vi "6_Eon.vi"(0 "file path (IN)":path, 1 "VGE":dbl, 2 "VCE":dbl, 5 "Project #":string, 7 "Request #":string, 9 "TEST #":string, 11 "error in (no error)":errorcluster) -> (4 "file path (OUT)":path, 6 "ON Region":waveform(dbl)[](graph) caption="Eon (uj)", 8 "Eon (uj)":dbl, 10 "DONE Eon":bool, 15 "error out":errorcluster)   [LabVIEW 2020]
uses:
  <vilib>/Waveform/WDTOps.llb/WDT Waveform Duration DBL.vi
  <vilib>/Waveform/WDTOps.llb/WDT Get Waveform Subset DBL.vi
  <vilib>/measure/mascope.llb/Transition Measurements 1 chan.vi
  <vilib>/measure/NI_MAPro.lvlib
panel:
  in  "Decision ?":bool
  in  "Cursor a : Channel 3\nfall edge tolerance":dbl=0.1
  in  "Cursor a : Channel 3\nfall edge number":i32=1 min=1
  in  "Cursor a : Channel 2\nrise edge tolerance":dbl=0.1
  in  "Cursor a : Channel 2\nrise edge number":i32=1 min=1
  out "Cursor a : Channel 2":dbl
  out "Cursor a : Channel 3":dbl
  out "Eon : XY Graph":cluster{"X":dbl, "Y":dbl}[](graph)
  out "Eon Area Y-axis":dbl[](array[numeric])
  out "Eon Area X-axis":dbl[](array[numeric])
  out "3% Vce":dbl
  out "10% Vge":dbl
  out "measurement info (CH3)":T1 {"ref levels"."ref units" items=["absolute", "relative"]; "ref levels"."high ref level" format="%.2p"; "ref levels"."low ref level" format="%.2p"; "ref levels"."mid ref level" format="%.2p"; "end time" format="%.6e"; "start time" format="%.6e"}
  out "measurement info (CH2)":T1 {"ref levels"."ref units" items=["absolute", "relative"]; "ref levels"."high ref level" format="%.2p"; "ref levels"."low ref level" format="%.2p"; "ref levels"."mid ref level" format="%.2p"; "end time" format="%.6e"; "start time" format="%.6e"}
  in  "reference  levels (CH2 initialize)":T2={"high ref level"=90.0, "mid ref level"=50.0, "low ref level"=10.0, "ref units"=1} {"ref units" items=["absolute", "percent"]; "high ref level" format="%0.2f"; "low ref level" format="%0.2f"; "mid ref level" format="%0.2f"}
  in  "reference  levels (CH3 initialize)":T2={"high ref level"=90.0, "mid ref level"=50.0, "low ref level"=10.0, "ref units"=1} {"ref units" items=["absolute", "percent"]; "high ref level" format="%0.2f"; "low ref level" format="%0.2f"; "mid ref level" format="%0.2f"}
  out "Waveform Graph":waveform(dbl)[](graph)
  # "From 10% Vge to 3% Vce"
  # "Default = 1"
  # "Default = 1"
  # "Default = 0.1"
  # "Default = 0.1"
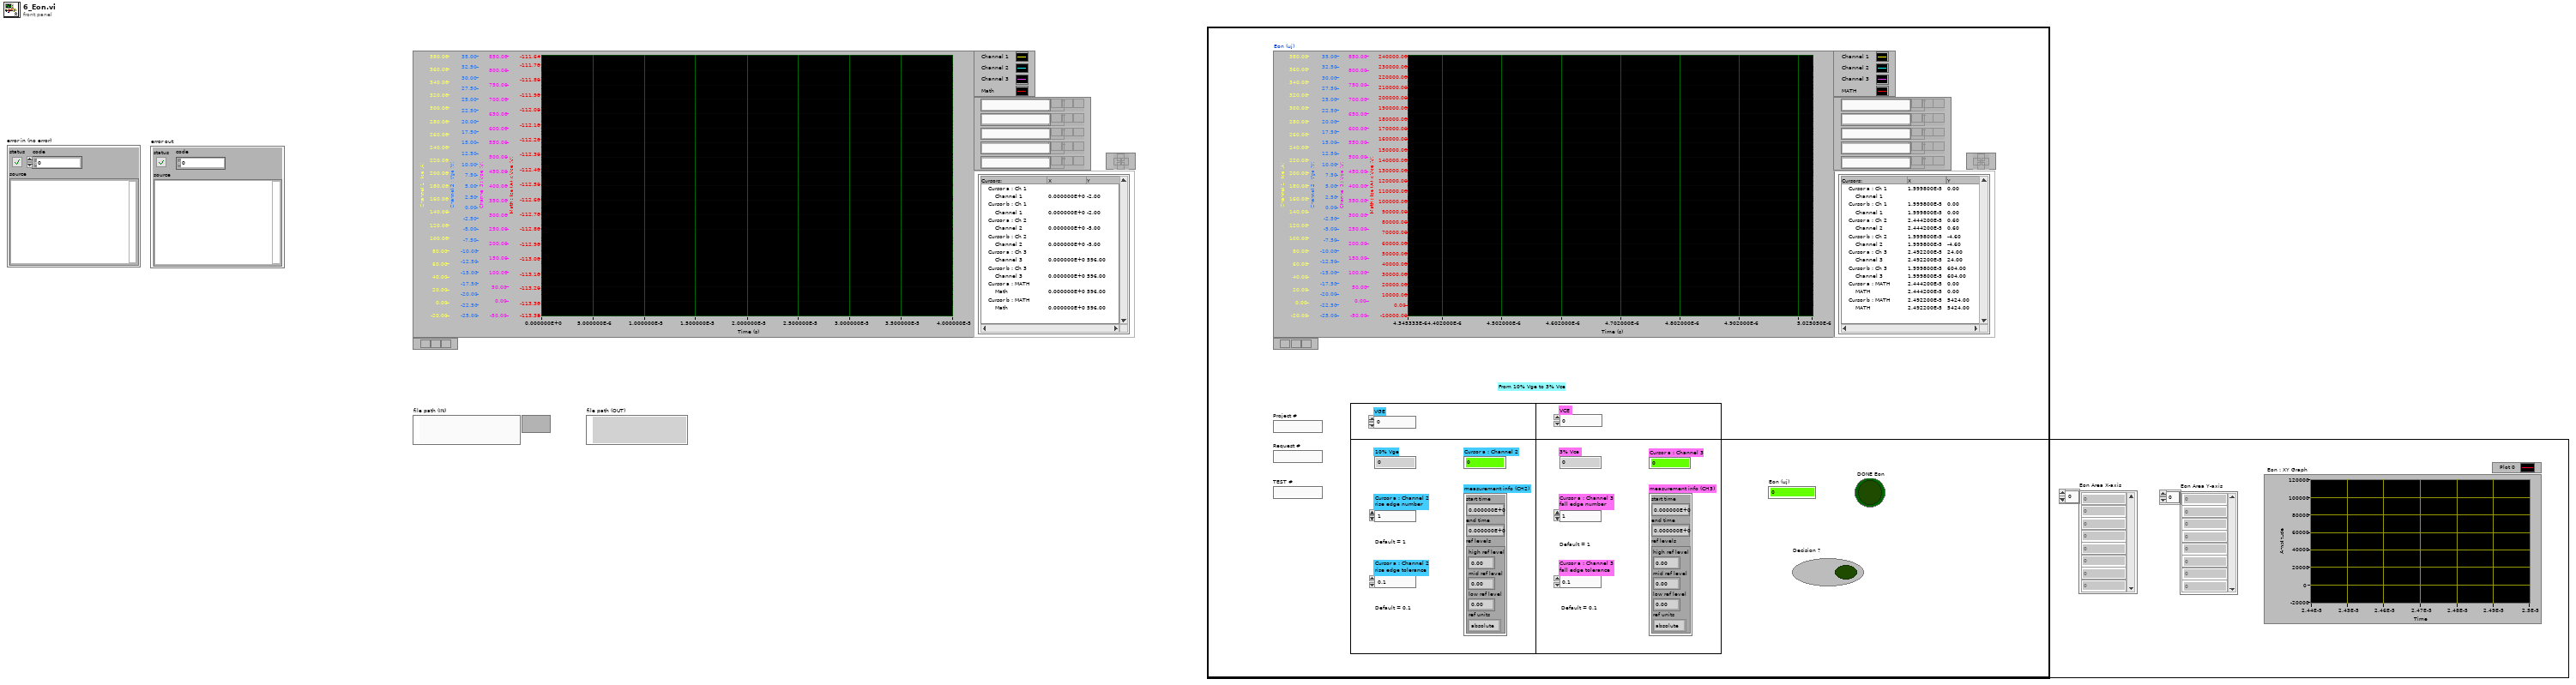
[diagram p1: front panel]
types:
  T1 = cluster{"start time":dbl, "end time":dbl, "ref levels":cluster{"high ref level":dbl, "mid ref level":dbl, "low ref level":dbl, "ref units":u16}}
  T2 = cluster{"high ref level":dbl, "mid ref level":dbl, "low ref level":dbl, "ref units":u16}
  T3 = enum32{"Invalid", "Standard", "Closed", "Hidden", "Minimized", "Maximized"}
  T4 = typedef "imagedata.ctl" = cluster{"image type":i32, "image depth":i32, "image":u8[], "mask":u8[], "colors":u32[], "Rectangle":cluster{"left":i16, "top":i16, "right":i16, "bottom":i16}}
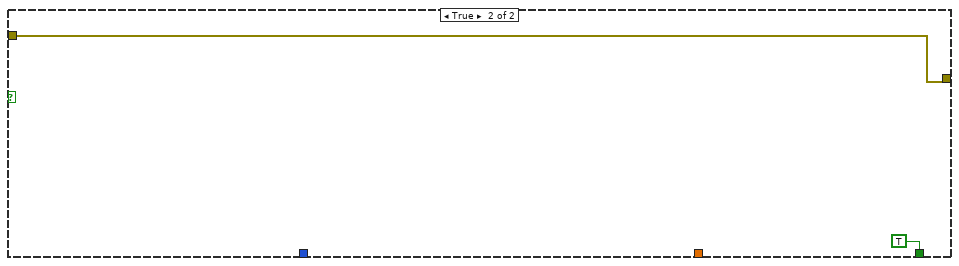
[diagram p6: hidden frame]
diagram:
  w7 = 0.0 ("Eon (uj)")
  w16 = errorcluster {"status"=FALSE, "code"=0, "source"=""} ("error out")
  w8 = FALSE ("DONE Tdon")
  w17 = waveform(dbl)[] [] ("Waveform Graph")
  n1 = local write "Eon (uj)"(w7) -> ()
  n2 = local write "Cursor a : Channel 2"(w7) -> ()
  n3 = local write "Cursor a : Channel 3"(w7) -> ()
  n4 = local write "Cursor a : Channel 2\nrise edge tolerance"(0.1 ("Cursor a : Channel 2\nrise edge tolerance")) -> ()
  n5 = local write "Cursor a : Channel 2\nrise edge number"(1 ("Cursor a : Channel 2\nrise edge number")) -> ()
  n6 = local write "DONE Eon"(w8) -> ()
  n7 = local write "Cursor a : Channel 3\nfall edge tolerance"(0.1 ("Cursor a : Channel 3\nfall edge tolerance")) -> ()
  n8 = local write "Cursor a : Channel 3\nfall edge number"(1 ("Cursor a : Channel 3\nfall edge number")) -> ()
  n9 = local write "Decision ?"(w8) -> ()
  n10 = local write "error out"(w16) -> ()
  n11 = local write "error in (no error)"(w16) -> ()
  n12 = local write "Waveform Graph"(w17) -> ()
  n13 = local write "ON Region"(w17) -> ()
  n14 = disable-structure shown="Disabled" {
    frame Disabled {
      n15 = control-ref of="This VI"() -> (w19:refnum<vi>)
      n16 = invoke class="VI" method="FP.Close"() -> (reference=w18:refnum<vi>)  [unwired: 2 in, 3 out]
      n17 = invoke class="VI" method="FP.Open"(reference=w19, "Activate"=TRUE ("Activate?"), "State"=T3."Maximized") -> (error in=w22:errorcluster, error out=w20:errorcluster)  [unwired: 1 in, 4 out]
      n18 = property class="VI"(reference=w19, error in=w20, "Front Panel.Closeable"=TRUE ("Front Panel Window:Closeable")) -> ()  [unwired: 2 out]
    }
    frame Enabled {
    }
  }
  n19 = flat-sequence {
    tunnel: ["file path (IN)"] -> w6
    tunnel: [w25] -> w5
    tunnel: [w36] -> w12
    tunnel: [w35] -> w9
    tunnel: w6 -> [w34]
    tunnel: w5 -> [w33]
    tunnel: w12 -> [w388]
    tunnel: [w387] -> w11
    tunnel: [w386] -> w10
    tunnel: w9 -> [w386]
    tunnel: w11 -> [w401]
    tunnel: w10 -> [w402]
    frame #0 {
      n20 = control-ref of="This VI"() -> (w27:refnum<vi>)
      n21 = invoke class="VI" method="FP.Open"(reference=w27, error in="error in (no error)", "Activate"=TRUE ("Activate?"), "State"=T3."Maximized") -> (error out=w28:errorcluster)  [unwired: 1 in, 4 out]
      n22 = property class="VI"(reference=w27, error in=w28, "Front Panel.Closeable"=TRUE ("Front Panel Window:Closeable")) -> (error out=w25:errorcluster)  [unwired: 1 out]
    }
    frame #1 {
      n23 = while {
        shift-right: [w43] -> w36
        shift-left: w33 -> [w41]
        tunnel: [w39] -> w35
        tunnel: w34 -> [w38]
        stop <- w44 stop-if-true
        n24 = flat-sequence {
          tunnel: w41 -> [w85]
          tunnel: [w85] -> w42
          tunnel: w38 -> [w78]
          tunnel: [w78] -> w37
          tunnel: [w117] -> w70
          tunnel: [w104] -> w69
          tunnel: [w115] -> w68
          tunnel: [w105] -> w67
          tunnel: [w87] -> w66
          tunnel: w42 -> [w191]
          tunnel: w37 -> [w186]
          tunnel: w70 -> [w231]
          tunnel: w69 -> [w230]
          tunnel: w68 -> [w229]
          tunnel: [w217] -> w65
          tunnel: w67 -> [w216]
          tunnel: [w216] -> w64
          tunnel: [w213] -> w63
          tunnel: [w212] -> w62
          tunnel: w66 -> [w211]
          tunnel: [w211] -> w61
          tunnel: w65 -> [w261]
          tunnel: [w258] -> w60
          tunnel: w64 -> [w267]
          tunnel: [w267] -> w59
          tunnel: w63 -> [w266]
          tunnel: [w266] -> w58
          tunnel: w62 -> [w265]
          tunnel: [w265] -> w57
          tunnel: w61 -> [w264]
          tunnel: [w264] -> w56
          tunnel: w60 -> [w278]
          tunnel: [w273] -> w55
          tunnel: w59 -> [w279]
          tunnel: [w279] -> w54
          tunnel: w58 -> [w269]
          tunnel: [w269] -> w53
          tunnel: w57 -> [w270]
          tunnel: [w270] -> w52
          tunnel: w56 -> [w277]
          tunnel: w55 -> [w360]
          tunnel: [w359] -> w51
          tunnel: w54 -> [w367]
          tunnel: [w367] -> w50
          tunnel: w53 -> [w356]
          tunnel: w52 -> [w355]
          tunnel: [w355] -> w49
          tunnel: [w356] -> w48
          tunnel: w51 -> [w378]
          tunnel: [w377] -> w47
          tunnel: w50 -> [w379]
          tunnel: [w379] -> w46
          tunnel: w49 -> [w372]
          tunnel: w48 -> [w371]
          tunnel: w47 -> [w382]
          tunnel: w46 -> [w380]
          tunnel: [w381] -> w45
          tunnel: [w380] -> w39
          frame #0 {
            w84 = waveform(dbl)[] [] ("Waveform Graph")
            w80 = 0.0 ("Eon (uj)")
            w79 = FALSE ("DONE Tdon")
            n25 = local write "Eon (uj)"(w80) -> ()
            n26 = local write "Cursor a : Channel 2"(w80) -> ()
            n27 = local write "Cursor a : Channel 3"(w80) -> ()
            n28 = local write "DONE Eon"(w79) -> ()
            n29 = local write "Decision ?"(w79) -> ()
            n30 = local write "Eon Area X-axis"(dbl[] [] ("Eon Area X-axis")) -> ()
            n31 = local write "Eon : XY Graph"(cluster{"X":dbl, "Y":dbl}[] [] ("Eon : XY Graph")) -> ()
            n32 = local write "Eon Area Y-axis"(dbl[] [] ("Eon Area X-axis")) -> ()
            n33 = Wait (ms)(milliseconds to wait=u32 200) -> ()  [unwired: 1 out]
            n34 = local write "Waveform Graph"(w84) -> ()
            n35 = local write "ON Region"(w84) -> ()
          }
          frame #1 {
            w94 = u16 1 items=["Samples", "Relative Time"] ("start/duration format")
            w168 = u16 1 items=["Samples", "Relative Time"] ("start/duration format")
            w178 = u16 1 items=["Samples", "Relative Time"] ("start/duration format")
            w179 = u16 1 items=["Samples", "Relative Time"] ("start/duration format")
            # "Channel 3"
            # "Channel 1"
            # "Channel MATH"
            # "MATH = Ch1 x Ch3"
            # "Channel 1"
            # "Channel 3"
            # "Channel 2"
            # "dt"
            # "Ch2"
            # "Ch1"
            n36 = call "3_ReadDatatoWaveform.vi"("error in (no error)"=w191, "file path (IN)"=w186) -> ("error out"=w164:errorcluster, "Waveform Graph"=→"Waveform Graph":waveform(dbl)[], "file path (OUT)"=w105:path, "dt"=w187:dbl, "Ch 2 Data"=w184:dbl[], "Ch 3 Data"=w188:dbl[], "Ch 1 Data"=w185:dbl[])  [unwired: 3 in]
            n37 = call <vilib>:"Beep.vi"("use system alert? (T)"=FALSE, "duration (msec)"=u32 200, "frequency (Hz)"=u32 2000) -> ()  [unwired: 9 in]
            n38 = To Time Stamp(1:0.0 ("number")) -> (0:w189:timestamp)
            n39 = disable-structure shown="Enabled" {
              disable-tunnel: w189 -> [w206 _]
              disable-tunnel: w187 -> [w205 _]
              disable-tunnel: w188 -> [w204 _]
              disable-tunnel: [w203 _] -> w101
              frame Enabled {
                # "Channel 3"
                n40 = Bundle By Name("Y"=w204, "dt"=w205, "t0"=w206) -> (w203:waveform(dbl))  [unwired: 1 in]
              }
              frame Disabled {
              }
            }
            n41 = disable-structure shown="Enabled" {
              disable-tunnel: w189 -> [w202 _]
              disable-tunnel: w187 -> [w201 _]
              disable-tunnel: w184 -> [w200 _]
              disable-tunnel: [w199 _] -> w167
              frame Enabled {
                # "Channel 2"
                n42 = Bundle By Name("Y"=w200, "dt"=w201, "t0"=w202) -> (w199:waveform(dbl))  [unwired: 1 in]
              }
              frame Disabled {
              }
            }
            n43 = disable-structure shown="Enabled" {
              disable-tunnel: w189 -> [w198 _]
              disable-tunnel: w187 -> [w197 _]
              disable-tunnel: w185 -> [w196 _]
              disable-tunnel: [w195 _] -> w102
              frame Enabled {
                # "Channel 1"
                n44 = Bundle By Name("Y"=w196, "dt"=w197, "t0"=w198) -> (w195:waveform(dbl))  [unwired: 1 in]
              }
              frame Disabled {
              }
            }
            n45 = Unbundle By Name(w101) -> ("Y"=w98:dbl[])
            n46 = Unbundle By Name(w102) -> ("Y"=w99:dbl[], "dt"=w86:dbl, "t0"=w100:timestamp)
            n47 = for {
              tunnel: w99 -> [w194] mode=indexing
              tunnel: w98 -> [w193] mode=indexing
              tunnel: [w192] -> w97 mode=indexing
              n48 = Multiply(x=w194, y=w193) -> (x*y=w192:dbl)
            }
            n49 = Bundle By Name("Y"=w97, "dt"=w86, "t0"=w100) -> (w89:waveform(dbl))  [unwired: 1 in]
            n50 = call-poly <vilib>:"Waveform Duration.vi"("waveform in"=w89) -> ("error out"=w90:errorcluster, "duration"=w92:dbl, "waveform out"=w95:waveform(dbl))  [unwired: 8 in]
            n51 = call-poly <vilib>:"Waveform Duration.vi"("error in (no error)"=w164, "waveform in"=w101) -> ("error out"=w172:errorcluster, "duration"=w170:dbl, "waveform out"=w103:waveform(dbl))  [unwired: 7 in]
            n52 = call-poly <vilib>:"Waveform Duration.vi"("error in (no error)"=w164, "waveform in"=w167) -> ("error out"=w173:errorcluster, "duration"=w176:dbl, "waveform out"=w174:waveform(dbl))  [unwired: 7 in]
            n53 = call-poly <vilib>:"Waveform Duration.vi"("error in (no error)"=w164, "waveform in"=w102) -> ("error out"=w183:errorcluster, "duration"=w180:dbl, "waveform out"=w182:waveform(dbl))  [unwired: 7 in]
            n54 = Divide(x=w92, y=2.0) -> (x/y=w93:dbl)
            n55 = Divide(x=w170, y=2.0) -> (x/y=w169:dbl)
            n56 = Divide(x=w176, y=2.0) -> (x/y=w177:dbl)
            n57 = Divide(x=w180, y=2.0) -> (x/y=w165:dbl)
            n58 = call-poly <vilib>:"Get Waveform Subset.vi"("start/duration format"=w94, "error in (no error)"=w90, "duration"=w93, "start samples/time"=w93, "waveform in"=w95) -> ("error out"=w88:errorcluster, "waveform out"=w87:waveform(dbl))  [unwired: 1 in, 2 out]
            n59 = call-poly <vilib>:"Get Waveform Subset.vi"("start/duration format"=w168, "error in (no error)"=w172, "duration"=w169, "start samples/time"=w169, "waveform in"=w103) -> ("error out"=w161:errorcluster, "waveform out"=w104:waveform(dbl))  [unwired: 1 in, 2 out]
            n60 = call-poly <vilib>:"Get Waveform Subset.vi"("start/duration format"=w178, "error in (no error)"=w173, "duration"=w177, "start samples/time"=w177, "waveform in"=w174) -> ("error out"=w162:errorcluster, "waveform out"=w117:waveform(dbl))  [unwired: 1 in, 2 out]
            n61 = call-poly <vilib>:"Get Waveform Subset.vi"("start/duration format"=w179, "error in (no error)"=w183, "duration"=w165, "start samples/time"=w165, "waveform in"=w182) -> ("error out"=w163:errorcluster, "waveform out"=w116:waveform(dbl))  [unwired: 1 in, 2 out]
            n62 = Build Array(w116, w117, w104, w87) -> (→"ON Region":waveform(dbl)[])
            n63 = Merge Errors(w163, w162, w161, w88) -> (w113:errorcluster)
            n64 = property on="ON Region" class="WFGraph (strict)"(error in=w113) -> (error out=w112:errorcluster, "Width"=w111:u32)  [unwired: 1 in, 1 out]
            n65 = property on="ON Region" class="WFGraph (strict)"(error in=w112, "Caption.Justify"=enum16{"Left", "Center", "Right"}."Left" ("Caption.Justification"), "Caption.Width"=w111, "Caption.FontBold"=TRUE ("Caption.Font:Bold"), "Caption.FontColor"=u32 16860 ("Caption.Font:Color"), "Caption.FontSize"=u32 24 ("Caption.Font:Size"), "Caption.Text"="Eon (uj)") -> (error out=w107:errorcluster)  [unwired: 1 in, 1 out]
            n66 = property on="ON Region" class="WFGraph (strict)"(error in=w107, "XScale.Offset"=w165) -> (error out=w141:errorcluster)  [unwired: 1 in, 1 out]
            n67 = property on="ON Region" class="WFGraph (strict)"(error in=w141, "Active Cursor"=u32 0, "Cursor.Cursor X"=0.0 ("Cursor.Cursor Position:Cursor X"), "Cursor.Cursor Y"=0.0 ("Cursor.Cursor Position:Cursor Y"), "Cursor.Visible"=FALSE) -> (error out=w140:errorcluster)  [unwired: 1 in, 1 out]
            n68 = property on="ON Region" class="WFGraph (strict)"(error in=w140, "Active Cursor"=u32 1, "Cursor.Cursor X"=0.0 ("Cursor.Cursor Position:Cursor X"), "Cursor.Cursor Y"=0.0 ("Cursor.Cursor Position:Cursor Y"), "Cursor.Visible"=FALSE) -> (error out=w139:errorcluster)  [unwired: 1 in, 1 out]
            n69 = property on="ON Region" class="WFGraph (strict)"(error in=w139, "Active Cursor"=u32 2, "Cursor.Cursor X"=0.0 ("Cursor.Cursor Position:Cursor X"), "Cursor.Cursor Y"=0.0 ("Cursor.Cursor Position:Cursor Y"), "Cursor.Visible"=FALSE) -> (error out=w138:errorcluster)  [unwired: 1 in, 1 out]
            n70 = property on="ON Region" class="WFGraph (strict)"(error in=w138, "Active Cursor"=u32 3, "Cursor.Cursor X"=0.0 ("Cursor.Cursor Position:Cursor X"), "Cursor.Cursor Y"=0.0 ("Cursor.Cursor Position:Cursor Y"), "Cursor.Visible"=FALSE) -> (error out=w121:errorcluster)  [unwired: 1 in, 1 out]
            n71 = property on="ON Region" class="WFGraph (strict)"(error in=w121, "Active Cursor"=u32 4, "Cursor.Cursor X"=0.0 ("Cursor.Cursor Position:Cursor X"), "Cursor.Cursor Y"=0.0 ("Cursor.Cursor Position:Cursor Y"), "Cursor.Visible"=FALSE) -> (error out=w120:errorcluster)  [unwired: 1 in, 1 out]
            n72 = property on="ON Region" class="WFGraph (strict)"(error in=w120, "Active Cursor"=u32 5, "Cursor.Cursor X"=0.0 ("Cursor.Cursor Position:Cursor X"), "Cursor.Cursor Y"=0.0 ("Cursor.Cursor Position:Cursor Y"), "Cursor.Visible"=FALSE) -> (error out=w119:errorcluster)  [unwired: 1 in, 1 out]
            n73 = property on="ON Region" class="WFGraph (strict)"(error in=w119, "Active Cursor"=u32 6, "Cursor.Cursor X"=0.0 ("Cursor.Cursor Position:Cursor X"), "Cursor.Cursor Y"=0.0 ("Cursor.Cursor Position:Cursor Y"), "Cursor.Visible"=FALSE) -> (error out=w118:errorcluster)  [unwired: 1 in, 1 out]
            n74 = property on="ON Region" class="WFGraph (strict)"(error in=w118, "Active Cursor"=u32 7, "Cursor.Cursor X"=0.0 ("Cursor.Cursor Position:Cursor X"), "Cursor.Cursor Y"=0.0 ("Cursor.Cursor Position:Cursor Y"), "Cursor.Visible"=FALSE) -> (error out=w115:errorcluster)  [unwired: 1 in, 1 out]
          }
          frame #2 {
            w246 = u16 1 items=["falling", "rising"] ("polarity (rising)")
            w247 = u16 0 items=["falling", "rising"] ("polarity (rising)")
            # "Cursor a : Channel 2"
            # "Cursor a : Channel 3"
            # "End Time 2nd Cursor"
            # "End Time 1st Cursor"
            # "2nd PARAMETER"
            # "Channel 3"
            # "1st PARAMETER"
            # "Channel 2"
            n75 = Divide(x=3.0, y=100.0) -> (x/y=w255:dbl)
            n76 = Divide(x=10.0, y=100.0) -> (x/y=w251:dbl)
            n77 = Multiply(x=w255, y="VCE") -> (x*y=w232:dbl)
            "3% Vce" <- w232
            n78 = Multiply(x=w251, y="VGE") -> (x*y=w239:dbl)
            "10% Vge" <- w239
            n79 = Add(x=w232, y="Cursor a : Channel 3\nfall edge tolerance") -> (x+y=w238:dbl)
            n80 = Subtract(x=w232, y="Cursor a : Channel 3\nfall edge tolerance") -> (x-y=w237:dbl)
            n81 = Add(x=w239, y="Cursor a : Channel 2\nrise edge tolerance") -> (x+y=w245:dbl)
            n82 = Subtract(x=w239, y="Cursor a : Channel 2\nrise edge tolerance") -> (x-y=w244:dbl)
            n83 = Bundle By Name(cluster="reference  levels (CH3 initialize)", "high ref level"=w238, "mid ref level"=w232, "low ref level"=w237, "ref units"=u16 0) -> (w234:T2)
            n84 = call-poly <vilib>:"Transition Measurements.vi"("edge number (1)"="Cursor a : Channel 3\nfall edge number", "error in (no error)"=w229, "reference levels"=w234, "polarity (rising)"=w247, "signal in"=w230) -> ("error out"=w226:errorcluster, "measurement info"=w233:T1)  [unwired: 1 in, 4 out]
            "measurement info (CH3)" <- w233
            n85 = Bundle By Name(cluster="reference  levels (CH2 initialize)", "high ref level"=w245, "mid ref level"=w239, "low ref level"=w244, "ref units"=u16 0) -> (w241:T2)
            n86 = call-poly <vilib>:"Transition Measurements.vi"("edge number (1)"="Cursor a : Channel 2\nrise edge number", "error in (no error)"=w229, "reference levels"=w241, "polarity (rising)"=w246, "signal in"=w231) -> ("error out"=w223:errorcluster, "measurement info"=w240:T1)  [unwired: 1 in, 4 out]
            "measurement info (CH2)" <- w240
            n87 = Unbundle By Name(w233) -> ("end time"=w213:dbl)
            n88 = Unbundle By Name(w240) -> ("end time"=w212:dbl)
            n89 = call <vilib>:"Beep.vi"("use system alert? (T)"=FALSE, "duration (msec)"=u32 200, "frequency (Hz)"=u32 2000) -> ()  [unwired: 9 in]
            n90 = property on="ON Region" class="WFGraph (strict)"(error in=w223, "Active Cursor"=u32 2, "Cursor.Cursor X"=w212, "Cursor.Visible"=TRUE, "Cursor.Cursor Name Visible"=TRUE) -> (error out=w218:errorcluster)  [unwired: 1 in, 1 out]
            n91 = property on="ON Region" class="WFGraph (strict)"(error in=w226, "Active Cursor"=u32 4, "Cursor.Cursor X"=w213, "Cursor.Visible"=TRUE, "Cursor.Cursor Name Visible"=TRUE) -> (error out=w219:errorcluster)  [unwired: 1 in, 1 out]
            n92 = Merge Errors(w219, w218) -> (w217:errorcluster)
          }
          frame #3 {
            # "Cursor a : Channel 3"
            # "Cursor a : Channel 2"
            n93 = property on="ON Region" class="WFGraph (strict)"(error in=w261, "Active Cursor"=u32 4) -> (error out=w260:errorcluster, "Cursor.Cursor Y"=→"Cursor a : Channel 3":dbl)  [unwired: 1 in, 1 out]
            n94 = property on="ON Region" class="WFGraph (strict)"(error in=w261, "Active Cursor"=u32 2) -> (error out=w259:errorcluster, "Cursor.Cursor Y"=→"Cursor a : Channel 2":dbl)  [unwired: 1 in, 1 out]
            n95 = Merge Errors(w260, w259) -> (w258:errorcluster)
          }
          frame #4 {
            # "https://forums.ni.com/t5/LabVIEW/area-under-curve-of-an-XY-graph-with-constant-non-equi-distant-x/m-p/254797?profile.language=en&query.id=125746#M137523"
            n96 = flat-sequence {
              tunnel: w278 -> [w285]
              tunnel: w269 -> [w284]
              tunnel: w270 -> [w283]
              tunnel: [w280] -> w276
              tunnel: w276 -> [w294]
              tunnel: w271 -> [w293]
              tunnel: [w292] -> w275
              tunnel: w275 -> [w338]
              tunnel: [w338] -> w274
              tunnel: [w336] -> w272
              tunnel: [w335] -> w268
              tunnel: [w354] -> w273
              tunnel: w274 -> [w354]
              tunnel: w272 -> [w344]
              tunnel: w268 -> [w345]
              frame #0 {
                # "Cursor b : MATH"
                # "Cursor a : MATH"
                n97 = property on="ON Region" class="WFGraph (strict)"(error in=w285, "Active Cursor"=u32 6, "Cursor.Cursor X"=w283, "Cursor.Visible"=TRUE, "Cursor.Cursor Name Visible"=TRUE) -> (error out=w281:errorcluster)  [unwired: 1 in, 1 out]
                n98 = property on="ON Region" class="WFGraph (strict)"(error in=w285, "Active Cursor"=u32 7, "Cursor.Cursor X"=w284, "Cursor.Visible"=TRUE, "Cursor.Cursor Name Visible"=TRUE) -> (error out=w282:errorcluster)  [unwired: 1 in, 1 out]
                n99 = Merge Errors(w282, w281) -> (w280:errorcluster)
              }
              frame #1 {
                n100 = while {
                  tunnel: w294 -> [w302]
                  tunnel: w293 -> [w299]
                  tunnel: [w296] -> w292
                  i -> [w301]
                  stop <- w303 stop-if-true
                  # "Cursor b : MATH"
                  # "Cursor a : MATH"
                  n101 = property on="ON Region" class="WFGraph (strict)"(error in=w302, "Active Cursor"=u32 7) -> (error out=w298:errorcluster, "Cursor.Cursor X"=w305:dbl)  [unwired: 1 in, 1 out]
                  n102 = property on="ON Region" class="WFGraph (strict)"(error in=w302, "Active Cursor"=u32 6) -> (error out=w300:errorcluster, "Cursor.Cursor X"=w307:dbl)  [unwired: 1 in, 1 out]
                  n103 = Merge Errors(w300, w298) -> (w297:errorcluster)
                  n104 = Equal?(x=w307, y=w305) -> (x = y?=w304:bool)
                  n105 = case shown="False" w304 {
                    tunnel: [FALSE ("Cursor.Visible") TRUE ("Cursor.Visible")] -> w303
                    tunnel: w301 -> [w313 _]
                    tunnel: w299 -> [w312 _]
                    tunnel: w297 -> [w311 w333]
                    tunnel: [w309 w333] -> w296
                    frame False {
                      n106 = flat-sequence {
                        tunnel: w313 -> [w319]
                        tunnel: w311 -> [w316]
                        tunnel: [w315] -> w310
                        tunnel: w312 -> [w329]
                        tunnel: w310 -> [w327]
                        tunnel: [w325] -> w309
                        frame #0 {
                          # "Cursor a : MATH"
                          n107 = property on="ON Region" class="WFGraph (strict)"(error in=w316, "Active Cursor"=u32 6) -> (error out=w315:errorcluster, "Cursor.Cursor X"=w318:dbl, "Cursor.Cursor Y"=w317:dbl)  [unwired: 1 in, 1 out]
                          n108 = local read "Eon Area Y-axis"() -> (w322:dbl[])
                          n109 = local read "Eon Area X-axis"() -> (w323:dbl[])
                          n110 = Insert Into Array(array=w322, index=w319, new element=w317) -> (w320:dbl[])
                          n111 = Insert Into Array(array=w323, index=w319, new element=w318) -> (w321:dbl[])
                          n112 = local write "Eon Area X-axis"(w321) -> ()
                          n113 = local write "Eon Area Y-axis"(w320) -> ()
                        }
                        frame #1 {
                          # "Cursor a : MATH"
                          # "Cursor a : MATH"
                          n114 = property on="ON Region" class="WFGraph (strict)"(error in=w327, "Active Cursor"=u32 6) -> (error out=w326:errorcluster, "Cursor.Cursor X"=w330:dbl)  [unwired: 1 in, 1 out]
                          n115 = Add(x=w330, y=w329) -> (x+y=w328:dbl)
                          n116 = property on="ON Region" class="WFGraph (strict)"(error in=w326, "Active Cursor"=u32 6, "Cursor.Cursor X"=w328) -> (error out=w325:errorcluster)  [unwired: 1 in, 1 out]
                        }
                      }
                    }
                    frame True {
                    }
                  }
                  n117 = Wait (ms)(milliseconds to wait=u32 1) -> ()  [unwired: 1 out]
                }
              }
              frame #2 {
                n118 = local read "Eon Area Y-axis"() -> (w335:dbl[])
                n119 = local read "Eon Area X-axis"() -> (w336:dbl[])
                n120 = Build Cluster Array(w336, w335) -> (w339:cluster{dbl, dbl}[])
                n121 = local write "Eon : XY Graph"(w339) -> ()
                n122 = Wait (ms)(milliseconds to wait=u32 50) -> ()  [unwired: 1 out]
              }
              frame #3 {
                n123 = Wait (ms)(milliseconds to wait=u32 50) -> ()  [unwired: 1 out]
                n124 = Delete From Array(array=w344, index=0) -> (array with subset deleted=w353:dbl[])  [unwired: 1 in, 1 out]
                n125 = Delete From Array(array=w345, index=0) -> (array with subset deleted=w347:dbl[])  [unwired: 1 in, 1 out]
                n126 = Subtract(x=w353, y=w344) -> (x-y=w352:dbl[])
                n127 = Add(x=w347, y=w345) -> (x+y=w351:dbl[])
                n128 = Compound Arithmetic op=MULTIPLY(w352, w351, invert 2.0 ("Numeric")) -> (w349:dbl[])
                n129 = Add Array Elements(numeric array=w349) -> (sum=w342:dbl)
                n130 = Multiply(x=w342, y=1000000.0) -> (x*y=→"Eon (uj)":dbl)
              }
            }
            n131 = Unbundle By Name(w277) -> ("dt"=w271:dbl)
          }
          frame #5 {
            # "Cursor a : MATH"
            # "Cursor b : MATH"
            n132 = property on="ON Region" class="WFGraph (strict)"(error in=w360, "Active Cursor"=u32 7, "Cursor.Cursor X"=w356, "Cursor.Visible"=TRUE, "Cursor.Cursor Name Visible"=TRUE) -> (error out=w357:errorcluster)  [unwired: 1 in, 1 out]
            n133 = property on="ON Region" class="WFGraph (strict)"(error in=w360, "Active Cursor"=u32 6, "Cursor.Cursor X"=w355, "Cursor.Visible"=TRUE, "Cursor.Cursor Name Visible"=TRUE) -> (error out=w358:errorcluster)  [unwired: 1 in, 1 out]
            n134 = Merge Errors(w357, w358) -> (w359:errorcluster)
          }
          frame #6 {
            # "2nd Cursor"
            # "1st Cursor"
            n135 = Subtract(x=w372, y=1e-07) -> (x-y=w374:dbl)
            n136 = Add(x=w371, y=1e-07) -> (x+y=w373:dbl)
            n137 = property on="ON Region" class="WFGraph (strict)"(error in=w378, "XScale.Minimum"=w374, "XScale.Maximum"=w373) -> (error out=w377:errorcluster)  [unwired: 1 in, 1 out]
            n138 = call <vilib>:"Beep.vi"("use system alert? (T)"=FALSE, "duration (msec)"=u32 200, "frequency (Hz)"=u32 2000) -> ()  [unwired: 9 in]
          }
          frame #7 {
            n139 = while {
              shift-right: [w383] -> w381
              shift-left: w382 -> [w383]
              stop <- "Decision ?" stop-if-true
              n140 = Wait (ms)(milliseconds to wait=u32 100) -> ()  [unwired: 1 out]
            }
          }
        }
        n141 = while {
          tunnel: [w72] -> w44
          shift-right: [w75] -> w43
          shift-left: w45 -> [w76]
          stop <- w74 stop-if-true
          n142 = Wait (ms)(milliseconds to wait=u32 100) -> ()  [unwired: 1 out]
          n143 = call "Display Message to User"("error in (no error)"=w76) -> ("error out"=w75:errorcluster, "NO"=w72:bool)  [unwired: 9 in]
          n144 = Or(x=w72, y=TRUE) -> (x .or. y?=w74:bool)
        }
        n145 = Wait (ms)(milliseconds to wait=u32 100) -> ()  [unwired: 1 out]
      }
    }
    frame #2 {
      w391 = "_"
      n146 = invoke on="ON Region" class="WFGraph (strict)" method="Get Image"(error in=w388) -> (error out=w394:errorcluster, "image data"=w397:T4)  [unwired: 5 in, 4 out]
      n147 = Concatenate Strings("C:\\Inductive_Switching_Project\\IndSw_Image\\" ("string"), "Project #", w391, "Request #", w391, "TEST #", w391, "Eon" ("string"), ".png" ("string")) -> (w398:string)
      n148 = String To Path(string=w398) -> (path=w396:path)
      n149 = call <vilib>:"Write PNG File.vi"("error in (no error)"=w394, "image data"=w397, "path to PNG file"=w396) -> ("error out"=w387:errorcluster)  [unwired: 7 in, 1 out]
      "DONE Eon" <- TRUE ("DONE Tdon")
    }
    frame #3 {
      n150 = disable-structure shown="Enabled" {
        disable-tunnel: w401 -> [w403 _]
        frame Enabled {
          n151 = control-ref of="This VI"() -> (w404:refnum<vi>)
          n152 = invoke class="VI" method="FP.Close"(reference=w404, error in=w403) -> ()  [unwired: 1 in, 3 out]
        }
        frame Disabled {
        }
      }
      "file path (OUT)" <- w402
      "error out" <- w401
    }
  }
  "Eon Area Y-axis" <- dbl[] [] ("Eon Area Y-axis")
  "Eon : XY Graph" <- cluster{"X":dbl, "Y":dbl}[] [] ("Eon : XY Graph")
  "Eon Area X-axis" <- dbl[] [] ("Eon Area X-axis")
